vi "P9374A NA Sweep single point frequency.vi"(6 "Data type":string(combo)="complex", 7 "Frequency Hz":dbl=1500000000.0, 8 "error in (no error)":errorcluster {"code" format="%.0x"}, 11 "instrument handle":refnum<k15>="P9374A") -> (0 "error out":errorcluster {"code" format="%.0x"}, 2 "Val":dbl[](array[numeric]) format="%.2e", 3 "instrument handle out":refnum<k15>="P9374A")   [LabVIEW 2021]
uses:
  <instrlib>/Agilent NA/Agilent NA.lvlib
panel:
  out "ValActualSize":i32=2
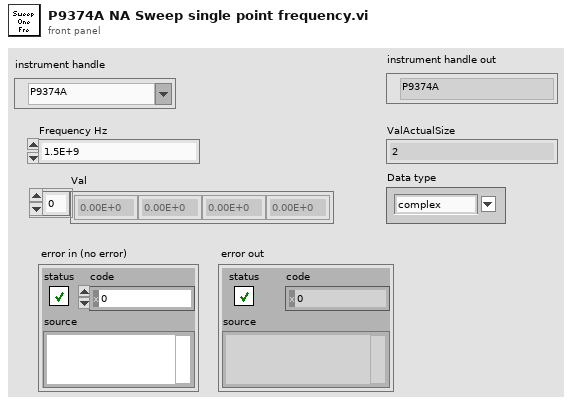
[diagram p1: front panel]
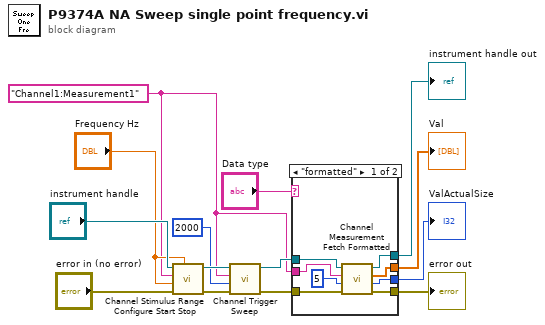
[diagram p0: block diagram]
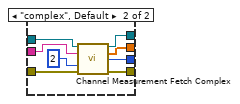
[diagram p2: hidden frame]
diagram:
  w6 = "Channel1:Measurement1" ("RepCapIdentifier")
  n1 = call <instrlib>:"Channel Stimulus Range Configure Start Stop.vi"("StopVal"="Frequency Hz", "error in (no error)"="error in (no error)", "StartVal"="Frequency Hz", "RepCapIdentifier"=w6, "instrument handle"="instrument handle") -> ("error out"=w9:errorcluster, "instrument handle out"=w11:refnum<k15>)  [unwired: 5 in]
  n2 = call <instrlib>:"Channel Trigger Sweep.vi"("error in (no error)"=w9, "TimeoutVal"=2000, "RepCapIdentifier"=w6, "instrument handle"=w11) -> ("error out"=w7:errorcluster, "instrument handle out"=w8:refnum<k15>)  [unwired: 6 in]
  n3 = case shown="\"formatted\"" "Data type" {
    tunnel: w8 -> [w22 w30]
    tunnel: w7 -> [w20 w29]
    tunnel: w6 -> [w21 w28]
    tunnel: [w18 w27] -> w5
    tunnel: [w17 w26] -> w4
    tunnel: [w15 w25] -> w3
    tunnel: [w16 w24] -> w2
    frame "formatted" {
      n4 = call <instrlib>:"Channel Measurement Fetch Formatted.vi"("error in (no error)"=w20, "RetValBufferSize"=5, "RepCapIdentifier"=w21, "instrument handle"=w22) -> ("error out"=w15:errorcluster, "RetValActualSize"=w16:i32, "RetVal"=w17:dbl[], "instrument handle out"=w18:refnum<k15>)  [unwired: 4 in]
    }
    frame "complex", Default {
      n5 = call <instrlib>:"Channel Measurement Fetch Complex.vi"("instrument handle"=w30, "RepCapIdentifier"=w28, "ValBufferSize"=2, "error in (no error)"=w29) -> ("instrument handle out"=w27:refnum<k15>, "Val"=w26:dbl[], "ValActualSize"=w24:i32, "error out"=w25:errorcluster)  [unwired: 8 in]
    }
  }
  "instrument handle out" <- w5
  "Val" <- w4
  "error out" <- w3
  "ValActualSize" <- w2
